vi "Test Sync.vi"() -> ()   [LabVIEW 2016]
uses:
  Hardware/Synchronization Device/Synchronization Device.lvclass
  C:/Program Files/National Instruments/LabVIEW 2016/vi.lib/ActorFramework/Actor/Actor.lvclass
  <vilib>/ActorFramework/Message Queue/Message Queue.lvclass/Message Queue.ctl
  <vilib>/ActorFramework/Message Enqueuer/Message Enqueuer.lvclass/Message Enqueuer.ctl
  <vilib>/ActorFramework/Message Enqueuer/Enqueue.vi
  <vilib>/ActorFramework/Stop Msg/Stop Msg.lvclass
  C:/Program Files/National Instruments/LabVIEW 2016/vi.lib/ActorFramework/Message/Message.lvclass
  <vilib>/ActorFramework/Message Priority Queue/Priority Enqueue.vi
  <vilib>/ActorFramework/Message Queue/Message Queue.lvclass
  <vilib>/ActorFramework/Actor/Actor.lvclass
panel:
  in  "Interval (ms)":dbl
  in  "Boolean":bool
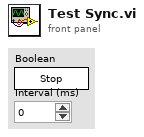
[diagram p1: front panel]
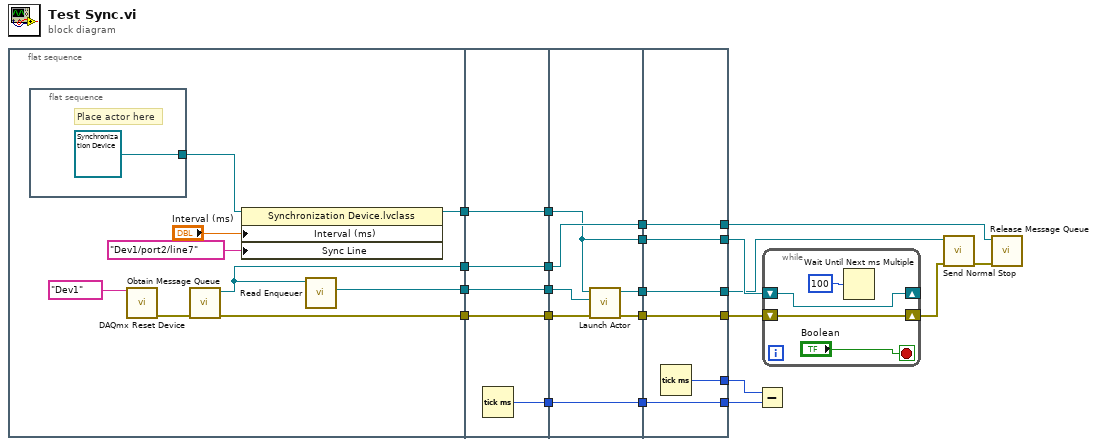
[diagram p0: block diagram]
diagram:
  n1 = flat-sequence {
    tunnel: [w31] -> w19
    tunnel: [w30] -> w18
    tunnel: [w29] -> w17
    tunnel: [w26] -> w16
    tunnel: w19 -> [w37]
    tunnel: w18 -> [w36]
    tunnel: w17 -> [w35]
    tunnel: w16 -> [w34]
    tunnel: [w37] -> w15
    tunnel: [w36] -> w14
    tunnel: [w35] -> w13
    tunnel: [w34] -> w12
    tunnel: [w33] -> w5
    tunnel: w15 -> [w44]
    tunnel: w14 -> [w43]
    tunnel: w13 -> [w41]
    tunnel: w12 -> [w42]
    tunnel: [w44] -> w9
    tunnel: [w40] -> w8
    tunnel: [w42] -> w7
    tunnel: [w39] -> w6
    tunnel: w5 -> [w39]
    tunnel: [w38] -> w2
    tunnel: [w48] -> w11
    tunnel: [w49] -> w10
    tunnel: [w50] -> w21
    tunnel: w9 -> [w50]
    tunnel: w8 -> [w49]
    tunnel: w7 -> [w48]
    tunnel: [w47] -> w3
    tunnel: w6 -> [w47]
    tunnel: [w46] -> w4
    tunnel: [w45] -> w1
    tunnel: w2 -> [w45]
    frame #0 {
      n2 = flat-sequence {
        tunnel: [refnum<class "Synchronization Device.lvclass"> refnum ("Synchronization Device.lvlib:Synchronization Device.lvclass")] -> w28
        frame #0 {
          # "Place actor here"
        }
      }
      n3 = call <vilib>:"DAQmx Reset Device.vi"("device in"=tag "Dev1") -> ("error out"=w25:errorcluster)  [unwired: 14 in]
      n4 = call <vilib>:"Obtain Message Queue.vi"("error in (no error)"=w25) -> ("error out"=w29:errorcluster, "Message Queue"=w31:refnum<class "Message Queue.lvclass">)  [unwired: 9 in]
      n5 = property class="Synchronization Device.lvclass"(reference=w28, "Interval (ms)"="Interval (ms)", "Sync Line"=tag "Dev1/port2/line7" ("lines")) -> (reference out=w26:refnum<class "Synchronization Device.lvclass">)  [unwired: 1 in, 1 out]
      n6 = call <vilib>:"Read Enqueuer.vi"("Message Queue"=w31) -> ("Message Enqueuer"=w30:refnum<class "Message Enqueuer.lvclass">)  [unwired: 10 in]
    }
    frame #1 {
      n7 = Tick Count (ms)() -> (millisecond timer value=w33:u32)
    }
    frame #2 {
      n8 = call <vilib>:"Launch Actor.vi"("error in (no error)"=w41, "Actor-to-Caller Enqueuer"=w43, "Actor"=w42) -> ("error out"=w40:errorcluster, "Caller-To-Actor Enqueuer"=w38:refnum<class "Message Enqueuer.lvclass">)  [unwired: 7 in]
    }
    frame #3 {
      n9 = Tick Count (ms)() -> (millisecond timer value=w46:u32)
    }
  }
  n10 = Subtract(x=w4, y=w3) -> ()  [unwired: 1 out]
  n11 = while {
    shift-right: [w53] -> w20
    shift-left: w10 -> [w53]
    shift-right: [w54] -> _
    shift-left: w11 -> [w54]
    stop <- "Boolean" stop-if-true
    n12 = Wait Until Next ms Multiple(millisecond multiple=u32 100) -> ()  [unwired: 1 out]
  }
  n13 = call <vilib>:"Send Normal Stop.vi"("error in (no error)"=w20, "Message Enqueuer"=w1) -> ("error out"=w22:errorcluster)  [unwired: 9 in]
  n14 = call <vilib>:"Release Message Queue.vi"("error in (no error)"=w22, "Message Queue"=w21) -> ()  [unwired: 8 in, 2 out]
